vi "test pin.vi"() -> ()   [LabVIEW 2020, in "PEU.lvlib" / "PEU.lvclass"]
uses:
  PEU.lvclass
panel:
  in  "Pin":u16
  in  "Link":cluster{"IP":string, "Port":u16}={"IP"="192.167.1.11", "Port"=4001}
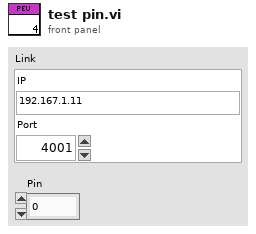
[diagram p1: front panel]
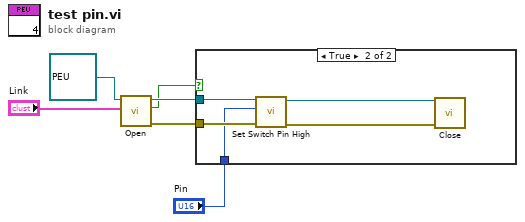
[diagram p0: block diagram]
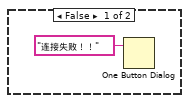
[diagram p2: hidden frame]
diagram:
  n1 = call "Open.vi"("Link"="Link", "PEU in"=refnum<class "PEU.lvclass"> refnum ("PEU.lvlib:PEU.lvclass")) -> ("error out"=w4:errorcluster, "Link_OK"=w1:bool, "PEU out"=w3:refnum<class "PEU.lvclass">)  [unwired: 7 in]
  n2 = case shown="True" w1 {
    tunnel: w4 -> [_ w12]
    tunnel: w3 -> [_ w11]
    tunnel: "Pin" -> [_ w8]
    frame False {
      n3 = One Button Dialog(message="连接失败！！") -> ()  [unwired: 1 in, 1 out]
    }
    frame True {
      n4 = call "Set Switch Pin High.vi"("error in (no error)"=w12, "Pin"=w8, "PEU in"=w11) -> ("error out"=w10:errorcluster, "PEU out"=w9:refnum<class "PEU.lvclass">)  [unwired: 7 in]
      n5 = call "Close.vi"("error in (no error)"=w10, "PEU in"=w9) -> ()  [unwired: 8 in, 2 out]
    }
  }
